vi "Notify Move In Previous Page.vi"(8 "error in (no error)":errorcluster, 10 "Test Channel Move In Previous":bool, 11 "Test Channel View in":refnum<class "Test Channel View.lvclass">) -> (0 "error out":errorcluster, 3 "Test Channel View out":refnum<class "Test Channel View.lvclass">)   [LabVIEW 2013, in "Test Channel View.lvlib" / "Test Channel View.lvclass"]
uses:
  Test Channel View.lvclass
  Test Channel View.lvclass/Test Channel View.ctl
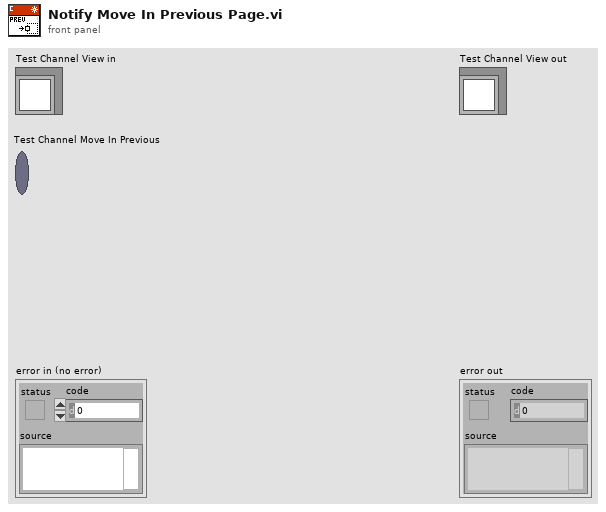
[diagram p1: front panel]
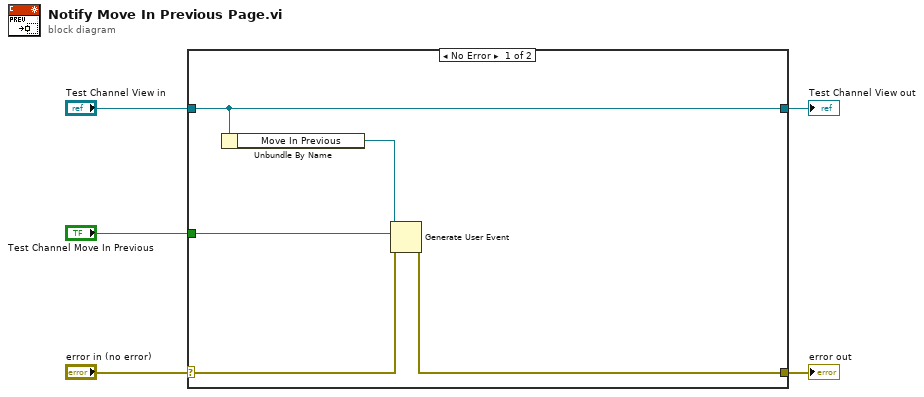
[diagram p0: block diagram]
diagram:
  n1 = case shown="No Error" "error in (no error)" {
    selector: "error in (no error)" -> [w7 w12]
    tunnel: [w6 w12] -> w4
    tunnel: [w10 w11] -> w2
    tunnel: "Test Channel View in" -> [w10 w11]
    tunnel: "Test Channel Move In Previous" -> [w8 _]
    frame No Error {
      n2 = Unbundle By Name(w10) -> ("Move In Previous"=w9:refnum<user-event>)
      n3 = Generate User Event(user event=w9, event data cluster=w8, error in=w7) -> (error out=w6:errorcluster)  [unwired: 1 in, 1 out]
    }
    frame Error {
    }
  }
  "error out" <- w4
  "Test Channel View out" <- w2
